vi "Hokuyo2LaserScan.vi"(4 "angle_max":dbl, 5 "range_max":dbl=5.6 format="%#_13g", 6 "angle_min":dbl, 7 "scan_time":dbl, 9 "Direction":dbl[](array[numeric]), 10 "Magnitude":dbl[](array[numeric]), 11 "frame_id":string) -> (3 "LaserScan":T1)   [LabVIEW 2014]
uses:
  Labview-ROS-Examples/Common/LaserScan.ctl
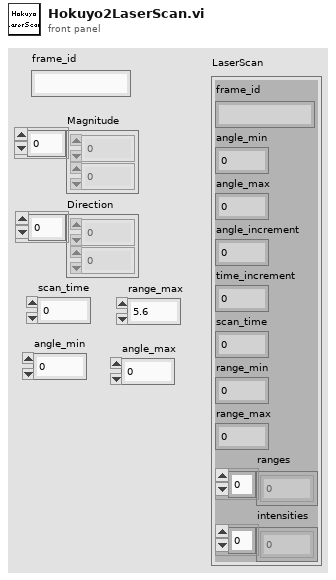
[diagram p1: front panel]
types:
  T1 = typedef "LaserScan.ctl" = cluster{"frame_id":string, "angle_min":dbl, "angle_max":dbl, "angle_increment":dbl, "time_increment":dbl, "scan_time":dbl, "range_min":dbl, "range_max":dbl, "ranges":dbl[], "intensities":dbl[]}
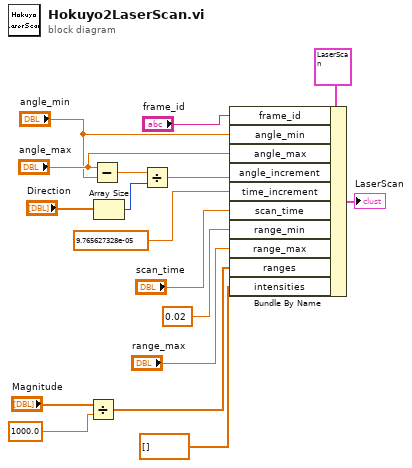
[diagram p0: block diagram]
diagram:
  n1 = Divide(x="Magnitude", y=1000.0) -> (x/y=w1:dbl[])
  n2 = Subtract(x="angle_max", y="angle_min") -> (x-y=w7:dbl)
  n3 = Array Size(array="Direction") -> (size(s)=w6:i32)
  n4 = Divide(x=w7, y=w6) -> (x/y=w5:dbl)
  n5 = Bundle By Name(cluster=T1 {"frame_id"="", "angle_min"=0.0, "angle_max"=0.0, "angle_increment"=0.0, "time_increment"=0.0, "scan_time"=0.0, "range_min"=0.0, "range_max"=0.0, "ranges"=[], "intensities"=[]} ("LaserScan"), "frame_id"="frame_id", "angle_min"="angle_min", "angle_max"="angle_max", "angle_increment"=w5, "time_increment"=9.765627328e-05, "scan_time"="scan_time", "range_min"=0.02, "range_max"="range_max", "ranges"=w1, "intensities"=dbl[] []) -> (→"LaserScan":T1)
